vi "Compile - Tx Buffered Channel Refs.vi"(6 "Packet Name":string, 7 "Timestamp Present?":bool, 8 "error in (no error)":errorcluster, 11 "Item Ref in":T1 format="%.0x") -> (0 "error out":errorcluster, 3 "Item Ref out":T1 format="%.0x", 4 "Tx Ref Array":T2(array[cluster]) {"VS Refs" format="%.0x"})   [LabVIEW 2016, in "UDP-Custom-Device System Explorer.lvlib"]
uses:
  UDP-Custom-Device System Explorer.lvlib
  Property Accessors/Tx Packet Accessors.lvlib
  <vilib>/NI Veristand/Custom Device API/Custom Device Item Ref.ctl
  <vilib>/NI VeriStand/Custom Device API/Custom Device API.lvlib
  Property Accessors/Buffered Data Packet.lvlib
  <vilib>/NI VeriStand/Custom Device Tools/Custom Device Utility Library/Custom Device Utility Library.lvlib
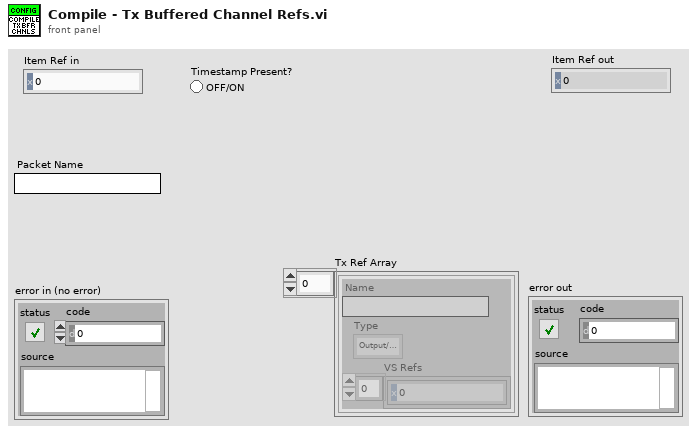
[diagram p1: front panel]
types:
  T1 = typedef "Custom Device API.lvlib/Custom Device Item Ref.ctl" = u64
  T2 = cluster{"Name":string, "Type":enum16{"Output/Write", "Input/Read", "Input/ReadWrite"}, "VS Refs":T1[]}[]
  T3 = cluster{"Name":string, "Type":enum16{"Output/Write", "Input/Read", "Input/ReadWrite"}, "VS Refs":T1[]}
  T4 = enum16{"Output/Write", "Input/Read", "Input/ReadWrite"}
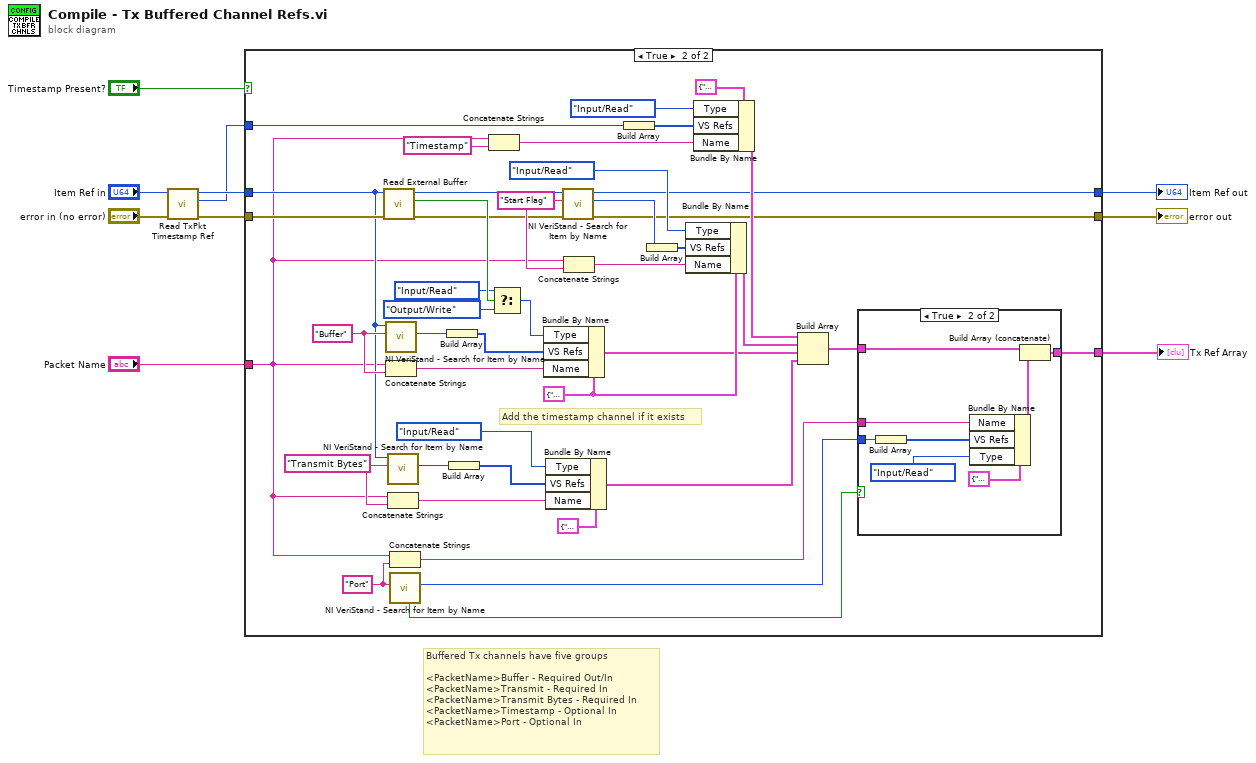
[diagram p0: block diagram]
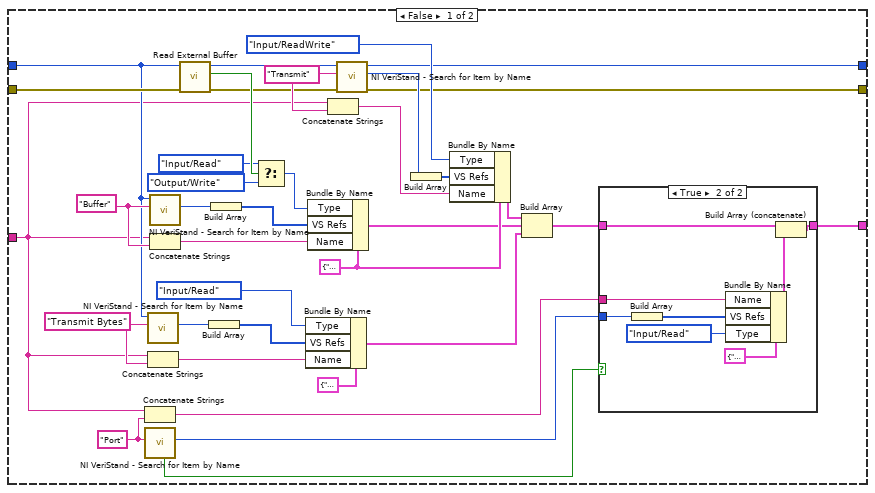
[diagram p2: hidden frame]
diagram:
  # "Buffered Tx channels have five groups\n\n<PacketName>Buffer - Required Out/In\n<PacketName>Transmit - Required In\n<PacketName>Transmit Bytes - Required In\n<PacketName>Timestamp - Optional In\n<PacketName>Port - Optional In"
  n1 = call "Read TxPkt Timestamp Ref.vi"("error in (no error)"="error in (no error)", "Node Ptr"="Item Ref in") -> ("error out"=w9:errorcluster, "Timestamp Ref"=w8:T1, "Node Ptr out"=w10:T1)  [unwired: 7 in]
  n2 = case shown="True" "Timestamp Present?" {
    tunnel: [w28 w73] -> w2
    tunnel: "Packet Name" -> [w14 w59]
    tunnel: [w16 w61] -> w1
    tunnel: w10 -> [w18 w63]
    tunnel: w9 -> [w46 w98]
    tunnel: w8 -> [_ w82]
    tunnel: [w30 w75] -> w3
    frame False {
      w15 = "Port" ("Item GUID")
      w24 = "Transmit Bytes" ("Item GUID")
      w32 = "Transmit" ("Item GUID")
      w27 = "Buffer" ("Item GUID")
      w36 = T3 {"Name"="", "Type"=enum."Output/Write", "VS Refs"=[]} ("Group")
      n3 = Concatenate Strings(w14, w15) -> (w12:string)
      n4 = call <vilib>:"NI VeriStand - Search for Item by Name.vi"("Item Name"=w15) -> ("Item Ref"=w11:T1, "Found"=w13:bool)  [unwired: 7 in, 2 out]
      n5 = call <vilib>:"NI VeriStand - Search for Item by Name.vi"("Item Name"=w24, "Section Ref in"=w18) -> ("Item Ref"=w25:T1)  [unwired: 6 in, 3 out]
      n6 = Concatenate Strings(w14, w24) -> (w21:string)
      n7 = call <vilib>:"NI VeriStand - Search for Item by Name.vi"("Item Name"=w27, "Section Ref in"=w18) -> ("Item Ref"=w26:T1)  [unwired: 6 in, 3 out]
      n8 = Concatenate Strings(w14, w27) -> (w45:string)
      n9 = call "Read External Buffer.vi"("error in (no error)"=w46, "Node Ptr"=w18) -> ("error out"=w31:errorcluster, "External Buffer"=w43:bool, "Node Ptr out"=w33:T1)  [unwired: 7 in]
      n10 = Build Array(w25) -> (w22:T1[])
      n11 = Build Array(w26) -> (w44:T1[])
      n12 = Select(t=T4."Input/Read" ("Type"), s=w43, f=T4."Output/Write" ("Type")) -> (s? t:f=w40:T4)
      n13 = Bundle By Name(cluster=T3 {"Name"="", "Type"=enum."Output/Write", "VS Refs"=[]} ("Group"), "Type"=T4."Input/Read", "VS Refs"=w22, "Name"=w21) -> (w20:T3)
      n14 = Bundle By Name(cluster=w36, "Type"=w40, "VS Refs"=w44, "Name"=w45) -> (w34:T3)
      n15 = Concatenate Strings(w14, w32) -> (w37:string)
      n16 = call <vilib>:"NI VeriStand - Search for Item by Name.vi"("error in"=w31, "Item Name"=w32, "Section Ref in"=w33) -> ("error out"=w28:errorcluster, "Item Ref"=w29:T1, "Section Ref out"=w30:T1)  [unwired: 5 in, 1 out]
      n17 = Build Array(w29) -> (w38:T1[])
      n18 = Bundle By Name(cluster=w36, "Type"=T4."Input/ReadWrite", "VS Refs"=w38, "Name"=w37) -> (w35:T3)
      n19 = Build Array(w35, w34, w20) -> (w17:T2)
      n20 = case shown="True" w13 {
        tunnel: w17 -> [w47 w55]
        tunnel: [w47 w54] -> w16
        tunnel: w11 -> [_ w51]
        tunnel: w12 -> [_ w49]
        frame False {
        }
        frame True {
          n21 = Build Array(w51) -> (w50:T1[])
          n22 = Bundle By Name(cluster=T3 {"Name"="", "Type"=enum."Output/Write", "VS Refs"=[]} ("Group"), "Name"=w49, "VS Refs"=w50, "Type"=T4."Input/Read") -> (w52:T3)
          n23 = Build Array (concatenate)(w55, w52) -> (w54:T2)
        }
      }
    }
    frame True {
      w60 = "Port" ("Item GUID")
      w64 = "Transmit Bytes" ("Item GUID")
      w77 = "Start Flag" ("Item GUID")
      w72 = "Buffer" ("Item GUID")
      w88 = T3 {"Name"="", "Type"=enum."Output/Write", "VS Refs"=[]} ("Group")
      # "Add the timestamp channel if it exists"
      n24 = call "Read External Buffer.vi"("error in (no error)"=w98, "Node Ptr"=w63) -> ("error out"=w76:errorcluster, "External Buffer"=w95:bool, "Node Ptr out"=w78:T1)  [unwired: 7 in]
      n25 = call <vilib>:"NI VeriStand - Search for Item by Name.vi"("Item Name"=w72, "Section Ref in"=w63) -> ("Item Ref"=w71:T1)  [unwired: 6 in, 3 out]
      n26 = Concatenate Strings(w59, w72) -> (w97:string)
      n27 = call <vilib>:"NI VeriStand - Search for Item by Name.vi"("Item Name"=w64, "Section Ref in"=w63) -> ("Item Ref"=w70:T1)  [unwired: 6 in, 3 out]
      n28 = Concatenate Strings(w59, w64) -> (w67:string)
      n29 = Concatenate Strings(w59, w60) -> (w57:string)
      n30 = call <vilib>:"NI VeriStand - Search for Item by Name.vi"("Item Name"=w60) -> ("Item Ref"=w56:T1, "Found"=w58:bool)  [unwired: 7 in, 2 out]
      n31 = Build Array(w71) -> (w96:T1[])
      n32 = Build Array(w70) -> (w68:T1[])
      n33 = Concatenate Strings(w59, "Timestamp" ("Item GUID")) -> (w83:string)
      n34 = Select(t=T4."Input/Read" ("Type"), s=w95, f=T4."Output/Write" ("Type")) -> (s? t:f=w92:T4)
      n35 = Bundle By Name(cluster=w88, "Type"=w92, "VS Refs"=w96, "Name"=w97) -> (w86:T3)
      n36 = Bundle By Name(cluster=T3 {"Name"="", "Type"=enum."Output/Write", "VS Refs"=[]} ("Group"), "Type"=T4."Input/Read", "VS Refs"=w68, "Name"=w67) -> (w65:T3)
      n37 = call <vilib>:"NI VeriStand - Search for Item by Name.vi"("error in"=w76, "Item Name"=w77, "Section Ref in"=w78) -> ("error out"=w73:errorcluster, "Item Ref"=w74:T1, "Section Ref out"=w75:T1)  [unwired: 5 in, 1 out]
      n38 = Concatenate Strings(w59, w77) -> (w89:string)
      n39 = Build Array(w82) -> (w84:T1[])
      n40 = Build Array(w74) -> (w90:T1[])
      n41 = Bundle By Name(cluster=w88, "Type"=T4."Input/Read", "VS Refs"=w90, "Name"=w89) -> (w87:T3)
      n42 = Bundle By Name(cluster=T3 {"Name"="", "Type"=enum."Output/Write", "VS Refs"=[]} ("Group"), "Type"=T4."Input/Read", "VS Refs"=w84, "Name"=w83) -> (w79:T3)
      n43 = Build Array(w79, w87, w86, w65) -> (w62:T2)
      n44 = case shown="True" w58 {
        tunnel: w62 -> [w99 w107]
        tunnel: [w99 w106] -> w61
        tunnel: w56 -> [_ w103]
        tunnel: w57 -> [_ w101]
        frame False {
        }
        frame True {
          n45 = Build Array(w103) -> (w102:T1[])
          n46 = Bundle By Name(cluster=T3 {"Name"="", "Type"=enum."Output/Write", "VS Refs"=[]} ("Group"), "Name"=w101, "VS Refs"=w102, "Type"=T4."Input/Read") -> (w104:T3)
          n47 = Build Array (concatenate)(w107, w104) -> (w106:T2)
        }
      }
    }
  }
  "Tx Ref Array" <- w1
  "error out" <- w2
  "Item Ref out" <- w3
